vi "Control_Loops Shift Variables.vi"(8 "error in":errorcluster, 11 "Main Config File Refnum":T1) -> (0 "error out":errorcluster, 3 "VARS Control_Loops":T2={"error"={"status"=FALSE, "code"=0, "source"=""}, "queue data"={"Command"="", "Variant Data"=variant}, "WDT Time Stamp 1"=timestamp(0 s since 1904-01-01), "Q_TO"=0, "LogErrors?"=FALSE, "Tag Set Directory"=path "c:/ni-rt/startup/tagset", "LogPath"=path "c:/ni-rt/startup/tagset", "PID Tag Sets"=[], "PIDChartRef"=refnum, "Loop SP-PVs"=[], "WDT_TO"=0} {"Loop SP-PVs"."Loop N" scale=0.0..100.0})   [LabVIEW 2018]
uses:
  Control_Loops Shift Variables.ctl
  Common/COMM_Queues/Command Queue Cluster.ctl
  Common/Controls/NGTS_PID Loop Tag and Gain Set.ctl
  <vilib>/Utility/config.llb/Config Data RefNum.ctl
  <vilib>/Utility/config.llb/NI_LVConfig.lvlib
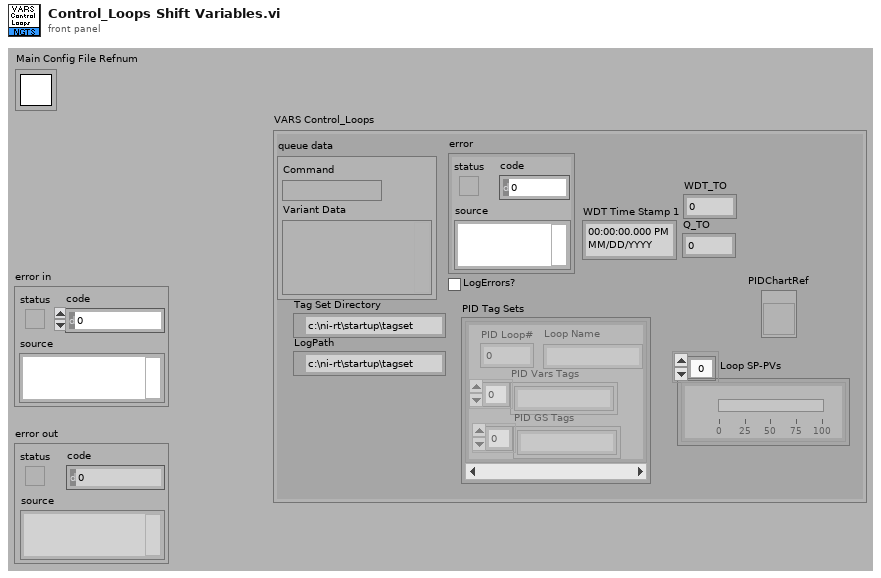
[diagram p1: front panel]
types:
  T1 = typedef "NI_LVConfig.lvlib/Config Data RefNum.ctl" = refnum<k1>
  T2 = typedef "Control_Loops Shift Variables.ctl" = cluster{"error":errorcluster, "queue data":T3, "WDT Time Stamp 1":timestamp, "Q_TO":i32, "LogErrors?":bool, "Tag Set Directory":path, "LogPath":path, "PID Tag Sets":T4[], "PIDChartRef":refnum<vi>, "Loop SP-PVs":cluster{"Loop N":cluster{dbl, dbl}, "Picture":picture}[], "WDT_TO":i32}
  T3 = typedef "Command Queue Cluster.ctl" = cluster{"Command":string, "Variant Data":variant}
  T4 = typedef "NGTS_PID Loop Tag and Gain Set.ctl" = cluster{"PID Loop#":i32, "PID Vars Tags":string[], "PID GS Tags":string[], "Loop Name":string}
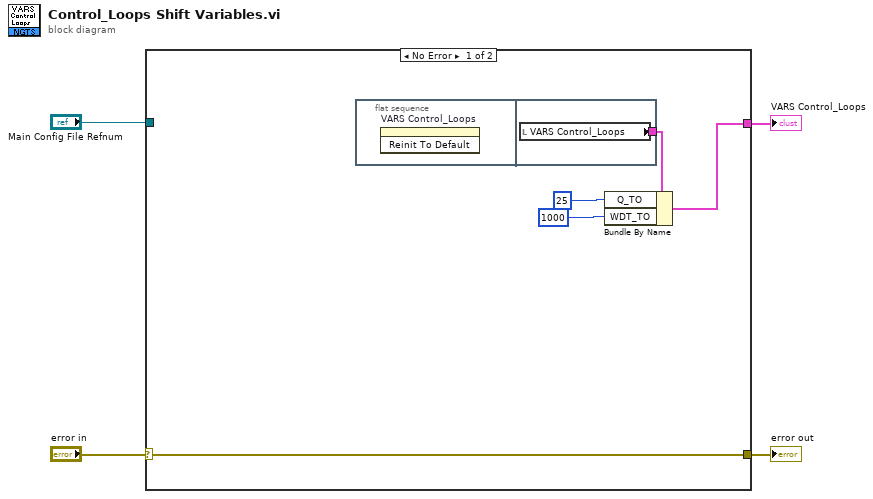
[diagram p0: block diagram]
diagram:
  n1 = case shown="No Error" "error in" {
    selector: "error in" -> [w8 w11]
    tunnel: [w9 _] -> w4
    tunnel: [w8 w11] -> w2
    tunnel: "Main Config File Refnum" -> [_ _]
    frame No Error {
      n2 = flat-sequence {
        tunnel: [w10] -> w6
        frame #0 {
          n3 = invoke on="VARS Control_Loops" class="Clust (strict)" method="Reinit To Default"() -> ()  [unwired: 3 in, 3 out]
        }
        frame #1 {
          n4 = local read "VARS Control_Loops"() -> (w10:T2)
        }
      }
      n5 = Bundle By Name(cluster=w6, "Q_TO"=25, "WDT_TO"=1000) -> (w9:T2)
    }
    frame Error {
    }
  }
  "VARS Control_Loops" <- w4
  "error out" <- w2
